vi "Configure Digital.vi"(0 "VISA resource name":refnum<visa-resource-name>, 5 "Binary Code (0 0 0)":u16(ring) items=["0 0 0", "0 0 1", "0 1 0 ", "0 1 1", "1 0 0", "1 0 1", "1 1 0", "1 1 1"], 11 "error in (no error)":errorcluster) -> (4 "VISA resource name out":refnum<visa-resource-name>, 15 "error out":errorcluster)   [LabVIEW 2012, in "Agilent 66XX Series.lvlib"]
doc: "This command sets the power supply digital control port when that port is configured for Digital I/O operation. Pin 3 in the back of the supply is the MSB. NOTE: Make sure that internal jumper has been adjusted. The power supply is shipped from factory in the FLT/INH mode and must be adjusted in order to operate as a general-purpose digital I/O port to control custom circuitry. If the hardware is not configured properly, this vi will generate an error."
uses:
  <instrlib>/Agilent 66XX Series/Agilent 66XX Series.lvlib
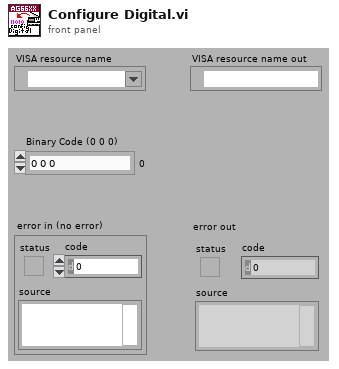
[diagram p1: front panel]
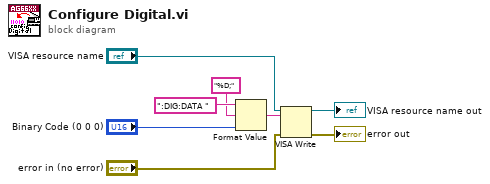
[diagram p0: block diagram]
diagram:
  n1 = Format Value(string ("")=":DIG:DATA ", format string="%D;", value (0)="Binary Code (0 0 0)") -> (output string=w5:string)
  n2 = VISA Write(VISA resource name="VISA resource name", write buffer=w5, error in (no error)="error in (no error)") -> (VISA resource name out=→"VISA resource name out":refnum<visa-resource-name>, error out=→"error out":errorcluster)  [unwired: 1 out]
